vi "GetDevices.vi"() -> ()   [LabVIEW 2018]
panel:
  out "devices":string[](array[string])
  out "error out":errorcluster
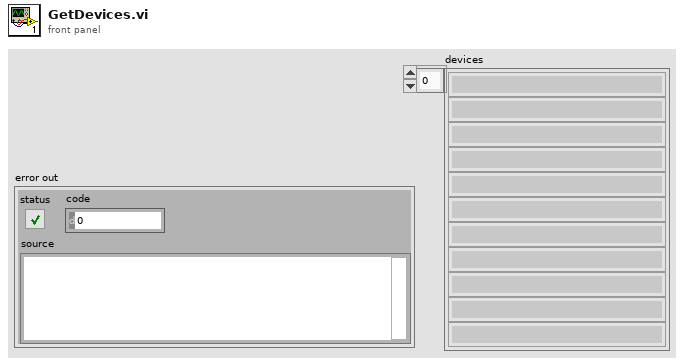
[diagram p1: front panel]
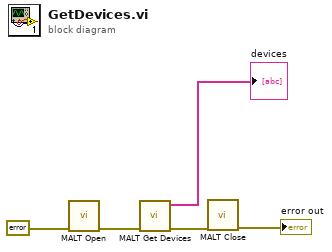
[diagram p0: block diagram]
diagram:
  n1 = call "MALT Open.vi"("error in"=errorcluster {"status"=FALSE, "code"=0, "source"=""}) -> ("error out"=w3:errorcluster)  [unwired: 10 in]
  n2 = call "MALT Get Devices.vi"("error in"=w3) -> ("error out"=w2:errorcluster, "devices"=→"devices":string[])  [unwired: 9 in]
  n3 = call "MALT Close.vi"("error in"=w2) -> ("error out"=→"error out":errorcluster)  [unwired: 10 in]
